vi "CAN_initialize2.vi"() -> (0 "Array 2":errorcluster[](array[cluster]), 1 "Array":refnum<class "sbCANopenBaseClass.lvclass">[](array[class]), 2 "Motors to use":bool[](array[boolean]))   [LabVIEW 2024]
uses:
  <vilib>/addons/Maxon Motor/EPOS2 CANopen/EPOS2 Library.lvlib
  <vilib>/addons/Maxon Motor/EPOS2 CANopen/EPOS2 Support Files/Polymorphic SubVIs/Config/EPOS2 Current Mode Configure.vi
  <vilib>/addons/Maxon Motor/EPOS2 CANopen/EPOS2 Support Files/Typedefs/EPOS2 Velocity Units.ctl
  <vilib>/addons/Maxon Motor/EPOS2 CANopen/EPOS2 Support Files/Typedefs/EPOS2 Config Data Input Current.ctl
  <vilib>/addons/Maxon Motor/EPOS2 CANopen/CANopen/CANopen IndCom Interface/sdCANopenIndCom.lvclass
  <vilib>/addons/Maxon Motor/EPOS2 CANopen/CANopen/sbCANopenBaseClass.lvclass
panel:
  out "MU":i32[](array[numeric])
  out "size(s) 3":i32
  out "appended array 2":refnum<class "sbCANopenBaseClass.lvclass">[](array[class])
  out "size(s)":i32
  out "size(s) 2":i32
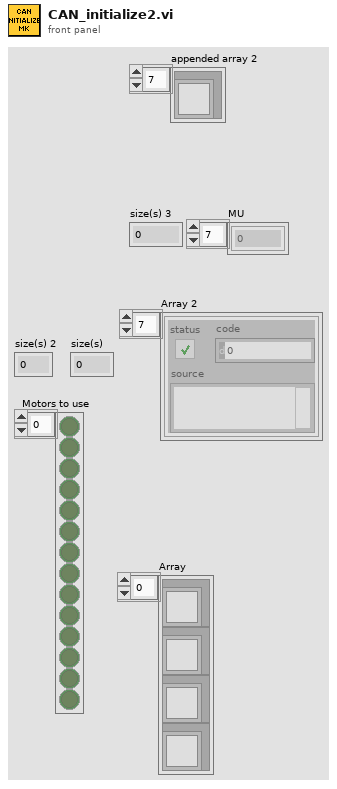
[diagram p1: front panel]
types:
  T1 = typedef "EPOS2 Library.lvlib/EPOS2 Config Data Input Current.ctl" = cluster{"Velocity Units":T2, "Max Velocity":i32}
  T2 = typedef "EPOS2 Library.lvlib/EPOS2 Velocity Units.ctl" = i8
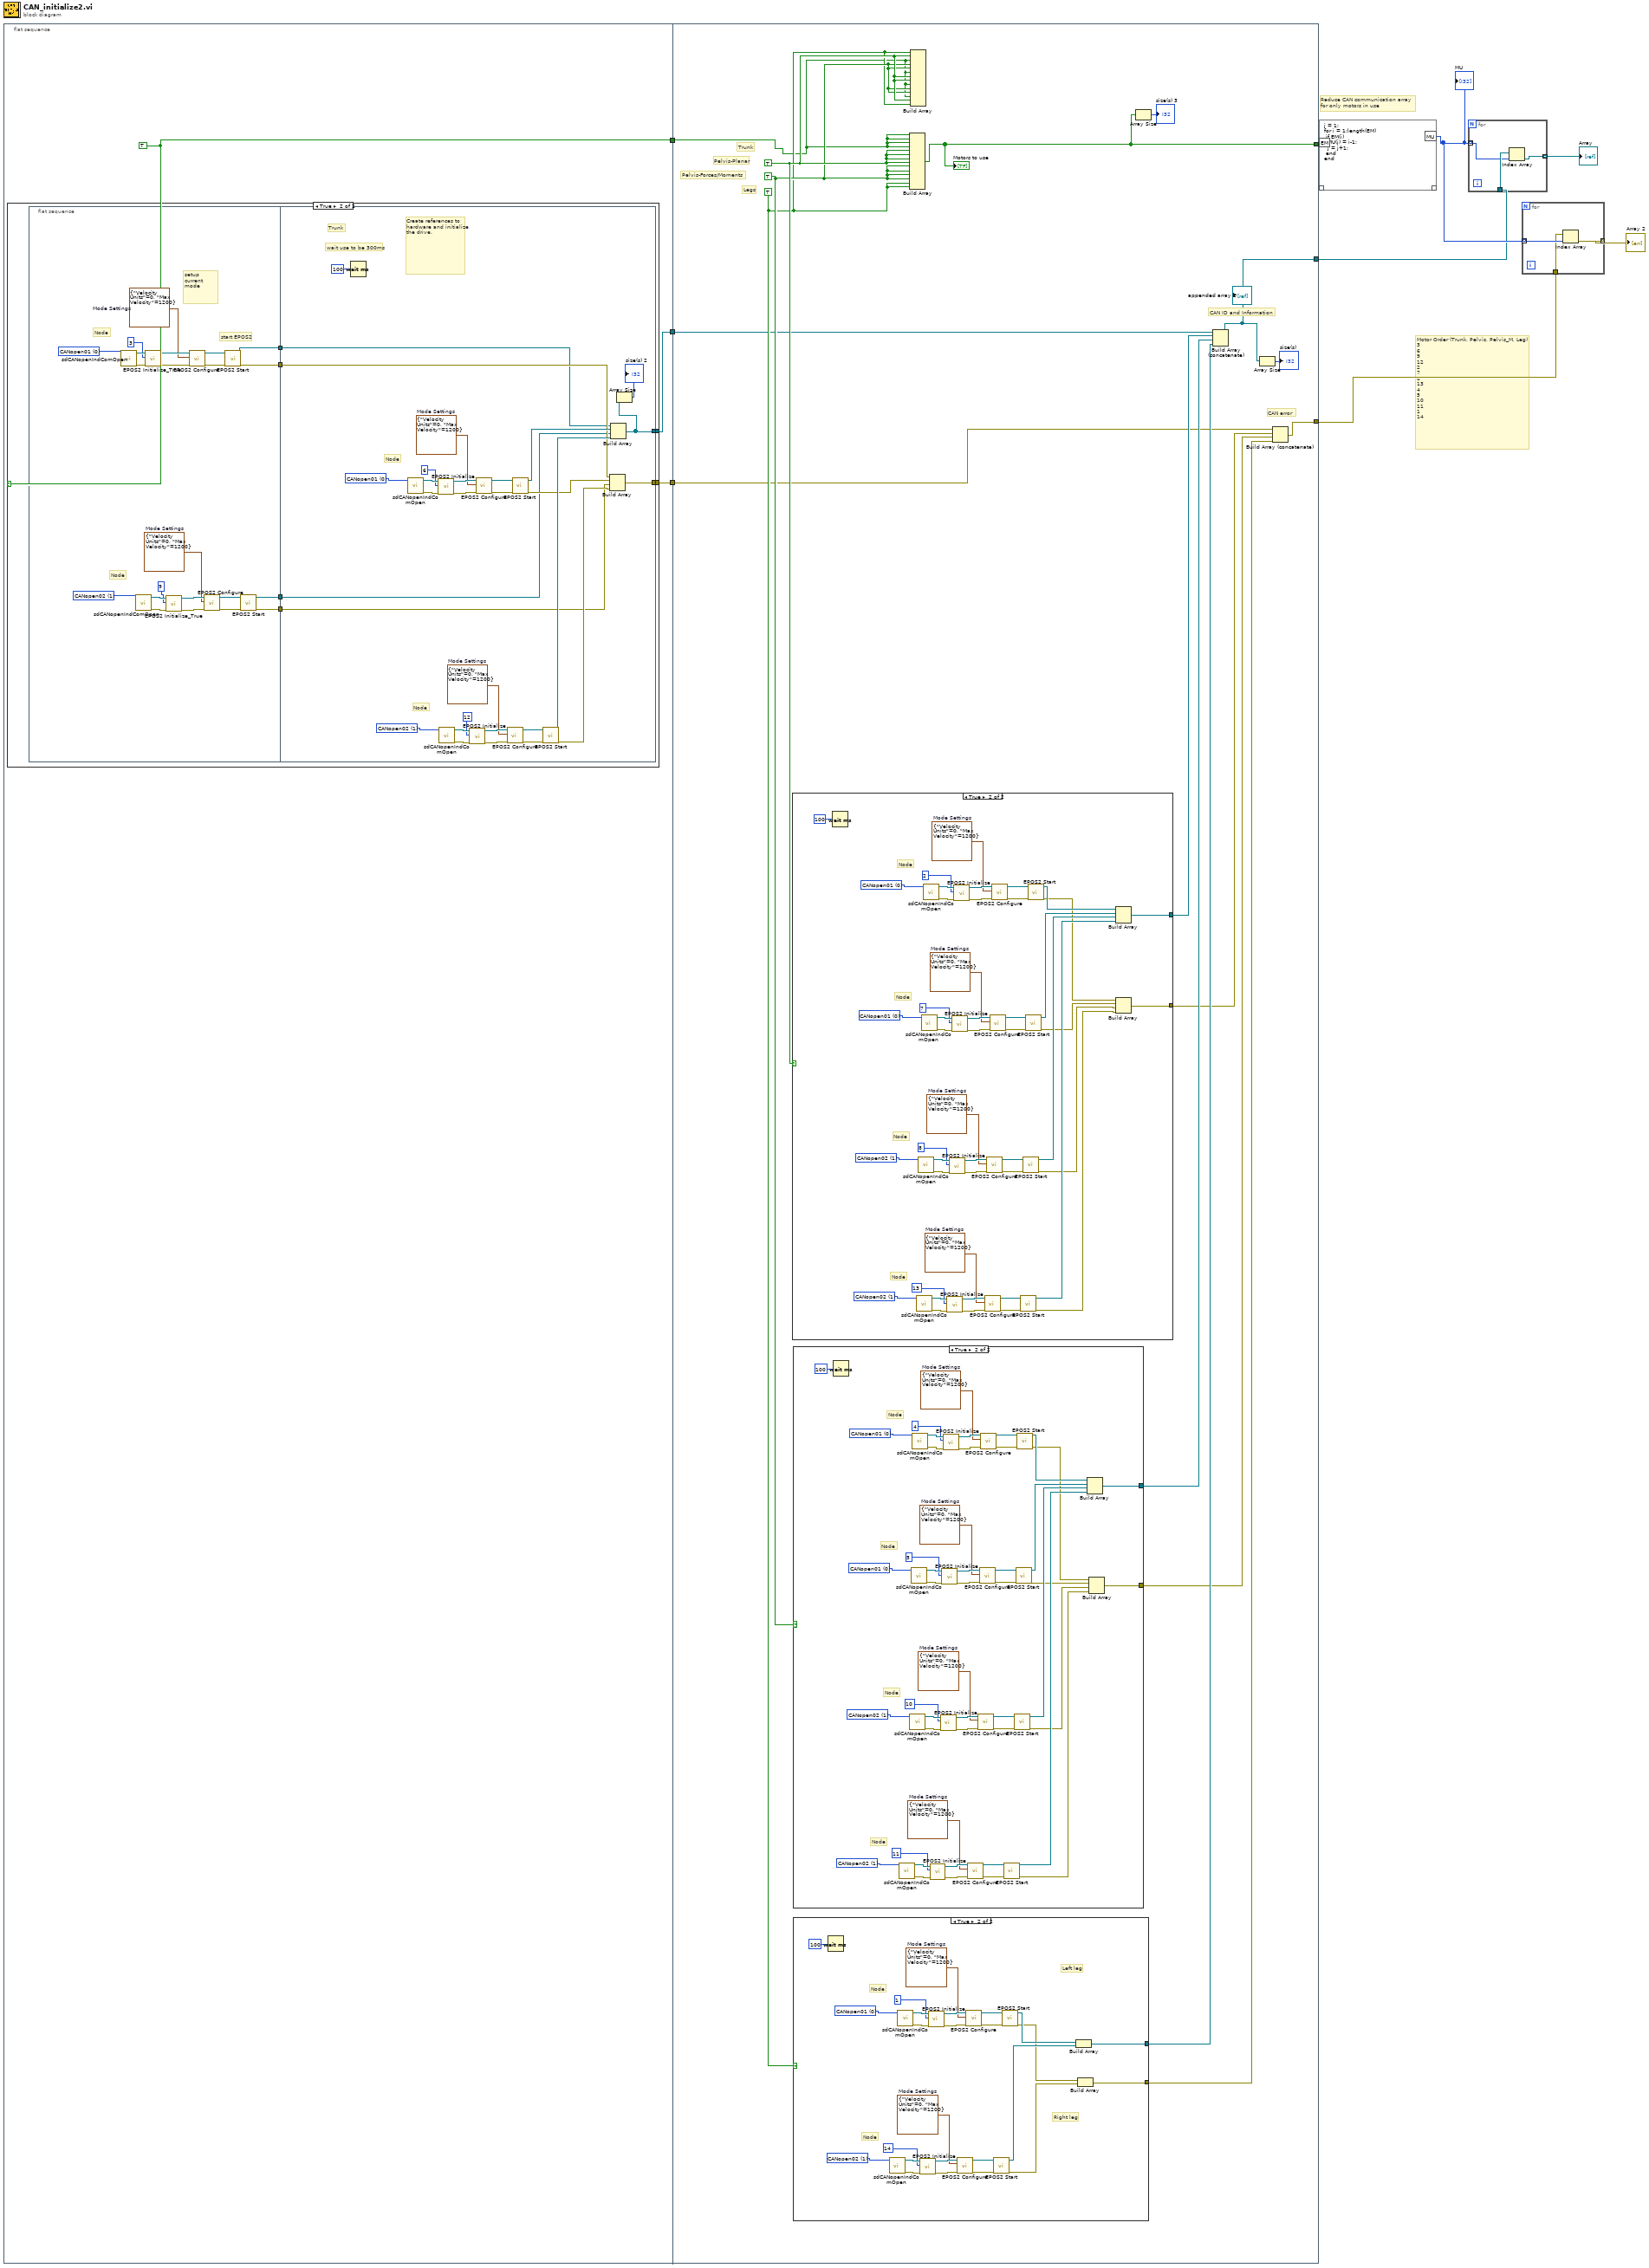
[diagram p0: block diagram]
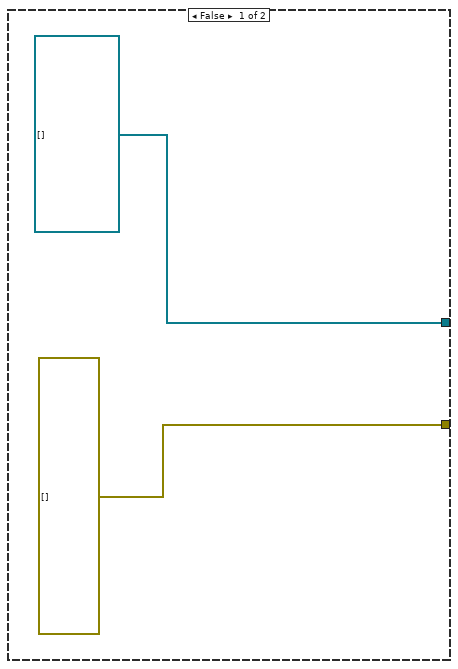
[diagram p2: hidden frame]
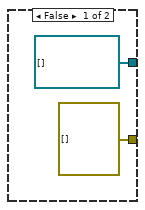
[diagram p3: hidden frame]
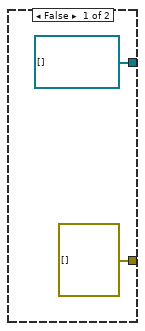
[diagram p4: hidden frame]
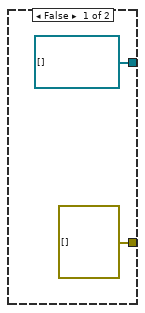
[diagram p5: hidden frame]
diagram:
  # "Motor Order (Trunk, Pelvis, Pelvis_M, Leg)\n3\n6\n9\n12\n2\n7\n8\n13\n4\n5\n10\n11\n1\n14"
  # "Reduce CAN communication array \nfor only motors in use"
  n1 = flat-sequence {
    tunnel: [w10] -> w3
    tunnel: [w12] -> w2
    tunnel: [w11] -> w1
    tunnel: [w82] -> w6
    tunnel: [w81] -> w5
    tunnel: [w76] -> w4
    tunnel: w3 -> [w75]
    tunnel: w2 -> [w74]
    tunnel: w1 -> [w73]
    frame #0 {
      w10 = TRUE
      n2 = case shown="True" w10 {
        tunnel: [refnum<class "sbCANopenBaseClass.lvclass">[] [] w20] -> w12
        tunnel: [errorcluster[] [] w19] -> w11
        frame False {
        }
        frame True {
          n3 = flat-sequence {
            tunnel: [w33] -> w18
            tunnel: [w32] -> w17
            tunnel: [w22] -> w16
            tunnel: [w21] -> w15
            tunnel: [w48] -> w20
            tunnel: [w47] -> w19
            tunnel: w18 -> [w46]
            tunnel: w17 -> [w45]
            tunnel: w16 -> [w44]
            tunnel: w15 -> [w43]
            frame #0 {
              w24 = u32 1 items=["CANopen01", "CANopen02", "CANopen03", "CANopen04", "CANopen05", "CANopen06", "CANopen07", "CANopen08", "CANopen09", "CANopen10", "CANopen11", "CANopen12", "CANopen13", "CANopen14", "CANopen15", "CANopen16", "CANopen17", "CANopen18", "CANopen19", "CANopen20", "CANopen21", "CANopen22", "CANopen23", "CANopen24", "CANopen25", "CANopen26", "CANopen27", "CANopen28", "CANopen29", "CANopen30", "CANopen31", "CANopen32"] ("Interface Name")
              w23 = T1 {"Velocity Units"=0, "Max Velocity"=1200}  # Mode Settings
              w35 = u32 0 items=["CANopen01", "CANopen02", "CANopen03", "CANopen04", "CANopen05", "CANopen06", "CANopen07", "CANopen08", "CANopen09", "CANopen10", "CANopen11", "CANopen12", "CANopen13", "CANopen14", "CANopen15", "CANopen16", "CANopen17", "CANopen18", "CANopen19", "CANopen20", "CANopen21", "CANopen22", "CANopen23", "CANopen24", "CANopen25", "CANopen26", "CANopen27", "CANopen28", "CANopen29", "CANopen30", "CANopen31", "CANopen32"] ("Interface Name")
              w34 = T1 {"Velocity Units"=0, "Max Velocity"=1200}  # Mode Settings
              # "Node"
              # "Node"
              # "start EPOS2"
              # "setup current mode"
              n4 = call <vilib>:"sdCANopenIndComOpen.vi"("Interface Name"=w35) -> ("error out"=w38:errorcluster, "SD CANopen Comm out"=w42:refnum<class "sbCANopenBaseClass.lvclass">)  [unwired: 9 in]
              n5 = call <vilib>:"sdCANopenIndComOpen.vi"("Interface Name"=w24) -> ("error out"=w27:errorcluster, "SD CANopen Comm out"=w31:refnum<class "sbCANopenBaseClass.lvclass">)  [unwired: 9 in]
              n6 = call <vilib>:"EPOS2 Initialize_True.vi"("error in"=w38, "Node ID"=u8 3, "CAN Session In"=w42) -> ("error out"=w37:errorcluster, "CANopen Session Out"=w40:refnum<class "sbCANopenBaseClass.lvclass">)  [unwired: 7 in]
              n7 = call <vilib>:"EPOS2 Initialize_True.vi"("error in"=w27, "Node ID"=u8 9, "CAN Session In"=w31) -> ("error out"=w26:errorcluster, "CANopen Session Out"=w29:refnum<class "sbCANopenBaseClass.lvclass">)  [unwired: 7 in]
              n8 = call-poly <vilib>:"EPOS2 Configure.vi"("error in"=w37, "Mode Settings"=w34, "CANopen Session In"=w40) -> ("error out"=w39:errorcluster, "CANopen Session Out"=w41:refnum<class "sbCANopenBaseClass.lvclass">)  [unwired: 7 in]
              n9 = call-poly <vilib>:"EPOS2 Configure.vi"("error in"=w26, "Mode Settings"=w23, "CANopen Session In"=w29) -> ("error out"=w28:errorcluster, "CANopen Session Out"=w30:refnum<class "sbCANopenBaseClass.lvclass">)  [unwired: 7 in]
              n10 = call <vilib>:"EPOS2 Start.vi"("error in"=w39, "CANopen Session In"=w41) -> ("error out"=w33:errorcluster, "CANopen Session Out"=w32:refnum<class "sbCANopenBaseClass.lvclass">)  [unwired: 8 in]
              n11 = call <vilib>:"EPOS2 Start.vi"("error in"=w28, "CANopen Session In"=w30) -> ("error out"=w22:errorcluster, "CANopen Session Out"=w21:refnum<class "sbCANopenBaseClass.lvclass">)  [unwired: 8 in]
            }
            frame #1 {
              w58 = u32 1 items=["CANopen01", "CANopen02", "CANopen03", "CANopen04", "CANopen05", "CANopen06", "CANopen07", "CANopen08", "CANopen09", "CANopen10", "CANopen11", "CANopen12", "CANopen13", "CANopen14", "CANopen15", "CANopen16", "CANopen17", "CANopen18", "CANopen19", "CANopen20", "CANopen21", "CANopen22", "CANopen23", "CANopen24", "CANopen25", "CANopen26", "CANopen27", "CANopen28", "CANopen29", "CANopen30", "CANopen31", "CANopen32"] ("Interface Name")
              w59 = T1 {"Velocity Units"=0, "Max Velocity"=1200}  # Mode Settings
              w66 = u32 0 items=["CANopen01", "CANopen02", "CANopen03", "CANopen04", "CANopen05", "CANopen06", "CANopen07", "CANopen08", "CANopen09", "CANopen10", "CANopen11", "CANopen12", "CANopen13", "CANopen14", "CANopen15", "CANopen16", "CANopen17", "CANopen18", "CANopen19", "CANopen20", "CANopen21", "CANopen22", "CANopen23", "CANopen24", "CANopen25", "CANopen26", "CANopen27", "CANopen28", "CANopen29", "CANopen30", "CANopen31", "CANopen32"] ("Interface Name")
              w67 = T1 {"Velocity Units"=0, "Max Velocity"=1200}  # Mode Settings
              # "wait use to be 300ms"
              # "Node"
              # "Node"
              # "Trunk"
              # "Create references to hardware and initialize the drive."
              n12 = Wait (ms)(milliseconds to wait=u32 100) -> ()  [unwired: 1 out]
              n13 = call <vilib>:"sdCANopenIndComOpen.vi"("Interface Name"=w66) -> ("error out"=w71:errorcluster, "SD CANopen Comm out"=w65:refnum<class "sbCANopenBaseClass.lvclass">)  [unwired: 9 in]
              n14 = call <vilib>:"EPOS2 Initialize.vi"("error in"=w71, "Node ID"=u8 6, "CAN Session In"=w65) -> ("error out"=w72:errorcluster, "CANopen Session Out"=w69:refnum<class "sbCANopenBaseClass.lvclass">)  [unwired: 1 in, 6 out]
              n15 = call <vilib>:"sdCANopenIndComOpen.vi"("Interface Name"=w58) -> ("error out"=w63:errorcluster, "SD CANopen Comm out"=w57:refnum<class "sbCANopenBaseClass.lvclass">)  [unwired: 9 in]
              n16 = call <vilib>:"EPOS2 Initialize.vi"("error in"=w63, "Node ID"=u8 12, "CAN Session In"=w57) -> ("error out"=w64:errorcluster, "CANopen Session Out"=w61:refnum<class "sbCANopenBaseClass.lvclass">)  [unwired: 1 in, 6 out]
              n17 = call-poly <vilib>:"EPOS2 Configure.vi"("error in"=w72, "Mode Settings"=w67, "CANopen Session In"=w69) -> ("error out"=w70:errorcluster, "CANopen Session Out"=w68:refnum<class "sbCANopenBaseClass.lvclass">)  [unwired: 7 in]
              n18 = call-poly <vilib>:"EPOS2 Configure.vi"("error in"=w64, "Mode Settings"=w59, "CANopen Session In"=w61) -> ("error out"=w62:errorcluster, "CANopen Session Out"=w60:refnum<class "sbCANopenBaseClass.lvclass">)  [unwired: 7 in]
              n19 = call <vilib>:"EPOS2 Start.vi"("error in"=w70, "CANopen Session In"=w68) -> ("error out"=w54:errorcluster, "CANopen Session Out"=w56:refnum<class "sbCANopenBaseClass.lvclass">)  [unwired: 8 in]
              n20 = call <vilib>:"EPOS2 Start.vi"("error in"=w62, "CANopen Session In"=w60) -> ("error out"=w53:errorcluster, "CANopen Session Out"=w55:refnum<class "sbCANopenBaseClass.lvclass">)  [unwired: 8 in]
              n21 = Build Array(w46, w54, w44, w53) -> (w47:errorcluster[])
              n22 = Build Array(w45, w56, w43, w55) -> (w48:refnum<class "sbCANopenBaseClass.lvclass">[])
              n23 = Array Size(array=w48) -> (size(s)=→"size(s) 2":i32)
            }
          }
        }
      }
    }
    frame #1 {
      w77 = TRUE
      w78 = TRUE
      w79 = TRUE
      # "CAN error"
      # "CAN ID and Information"
      # "Legs"
      # "Pelvis-Forces/Moments"
      # "Pelvis-Planar"
      # "Trunk"
      n24 = case shown="True" w79 {
        tunnel: [refnum<class "sbCANopenBaseClass.lvclass">[] [] w178] -> w89
        tunnel: [errorcluster[] [] w173] -> w86
        frame False {
        }
        frame True {
          w184 = u32 1 items=["CANopen01", "CANopen02", "CANopen03", "CANopen04", "CANopen05", "CANopen06", "CANopen07", "CANopen08", "CANopen09", "CANopen10", "CANopen11", "CANopen12", "CANopen13", "CANopen14", "CANopen15", "CANopen16", "CANopen17", "CANopen18", "CANopen19", "CANopen20", "CANopen21", "CANopen22", "CANopen23", "CANopen24", "CANopen25", "CANopen26", "CANopen27", "CANopen28", "CANopen29", "CANopen30", "CANopen31", "CANopen32"] ("Interface Name")
          w185 = T1 {"Velocity Units"=0, "Max Velocity"=1200}  # Mode Settings
          w192 = u32 1 items=["CANopen01", "CANopen02", "CANopen03", "CANopen04", "CANopen05", "CANopen06", "CANopen07", "CANopen08", "CANopen09", "CANopen10", "CANopen11", "CANopen12", "CANopen13", "CANopen14", "CANopen15", "CANopen16", "CANopen17", "CANopen18", "CANopen19", "CANopen20", "CANopen21", "CANopen22", "CANopen23", "CANopen24", "CANopen25", "CANopen26", "CANopen27", "CANopen28", "CANopen29", "CANopen30", "CANopen31", "CANopen32"] ("Interface Name")
          w193 = T1 {"Velocity Units"=0, "Max Velocity"=1200}  # Mode Settings
          w200 = u32 0 items=["CANopen01", "CANopen02", "CANopen03", "CANopen04", "CANopen05", "CANopen06", "CANopen07", "CANopen08", "CANopen09", "CANopen10", "CANopen11", "CANopen12", "CANopen13", "CANopen14", "CANopen15", "CANopen16", "CANopen17", "CANopen18", "CANopen19", "CANopen20", "CANopen21", "CANopen22", "CANopen23", "CANopen24", "CANopen25", "CANopen26", "CANopen27", "CANopen28", "CANopen29", "CANopen30", "CANopen31", "CANopen32"] ("Interface Name")
          w201 = T1 {"Velocity Units"=0, "Max Velocity"=1200}  # Mode Settings
          w208 = u32 0 items=["CANopen01", "CANopen02", "CANopen03", "CANopen04", "CANopen05", "CANopen06", "CANopen07", "CANopen08", "CANopen09", "CANopen10", "CANopen11", "CANopen12", "CANopen13", "CANopen14", "CANopen15", "CANopen16", "CANopen17", "CANopen18", "CANopen19", "CANopen20", "CANopen21", "CANopen22", "CANopen23", "CANopen24", "CANopen25", "CANopen26", "CANopen27", "CANopen28", "CANopen29", "CANopen30", "CANopen31", "CANopen32"] ("Interface Name")
          w209 = T1 {"Velocity Units"=0, "Max Velocity"=1200}  # Mode Settings
          # "Node"
          # "Node"
          # "Node"
          # "Node"
          n25 = Wait (ms)(milliseconds to wait=u32 100) -> ()  [unwired: 1 out]
          n26 = call <vilib>:"sdCANopenIndComOpen.vi"("Interface Name"=w184) -> ("error out"=w189:errorcluster, "SD CANopen Comm out"=w183:refnum<class "sbCANopenBaseClass.lvclass">)  [unwired: 9 in]
          n27 = call <vilib>:"sdCANopenIndComOpen.vi"("Interface Name"=w192) -> ("error out"=w197:errorcluster, "SD CANopen Comm out"=w191:refnum<class "sbCANopenBaseClass.lvclass">)  [unwired: 9 in]
          n28 = call <vilib>:"sdCANopenIndComOpen.vi"("Interface Name"=w200) -> ("error out"=w205:errorcluster, "SD CANopen Comm out"=w199:refnum<class "sbCANopenBaseClass.lvclass">)  [unwired: 9 in]
          n29 = call <vilib>:"sdCANopenIndComOpen.vi"("Interface Name"=w208) -> ("error out"=w213:errorcluster, "SD CANopen Comm out"=w207:refnum<class "sbCANopenBaseClass.lvclass">)  [unwired: 9 in]
          n30 = call <vilib>:"EPOS2 Initialize.vi"("error in"=w189, "Node ID"=u8 13, "CAN Session In"=w183) -> ("error out"=w190:errorcluster, "CANopen Session Out"=w187:refnum<class "sbCANopenBaseClass.lvclass">)  [unwired: 1 in, 6 out]
          n31 = call <vilib>:"EPOS2 Initialize.vi"("error in"=w197, "Node ID"=u8 8, "CAN Session In"=w191) -> ("error out"=w198:errorcluster, "CANopen Session Out"=w195:refnum<class "sbCANopenBaseClass.lvclass">)  [unwired: 1 in, 6 out]
          n32 = call <vilib>:"EPOS2 Initialize.vi"("error in"=w205, "Node ID"=u8 7, "CAN Session In"=w199) -> ("error out"=w206:errorcluster, "CANopen Session Out"=w203:refnum<class "sbCANopenBaseClass.lvclass">)  [unwired: 1 in, 6 out]
          n33 = call <vilib>:"EPOS2 Initialize.vi"("error in"=w213, "Node ID"=u8 2, "CAN Session In"=w207) -> ("error out"=w214:errorcluster, "CANopen Session Out"=w211:refnum<class "sbCANopenBaseClass.lvclass">)  [unwired: 1 in, 6 out]
          n34 = call-poly <vilib>:"EPOS2 Configure.vi"("error in"=w190, "Mode Settings"=w185, "CANopen Session In"=w187) -> ("error out"=w188:errorcluster, "CANopen Session Out"=w186:refnum<class "sbCANopenBaseClass.lvclass">)  [unwired: 7 in]
          n35 = call-poly <vilib>:"EPOS2 Configure.vi"("error in"=w198, "Mode Settings"=w193, "CANopen Session In"=w195) -> ("error out"=w196:errorcluster, "CANopen Session Out"=w194:refnum<class "sbCANopenBaseClass.lvclass">)  [unwired: 7 in]
          n36 = call-poly <vilib>:"EPOS2 Configure.vi"("error in"=w206, "Mode Settings"=w201, "CANopen Session In"=w203) -> ("error out"=w204:errorcluster, "CANopen Session Out"=w202:refnum<class "sbCANopenBaseClass.lvclass">)  [unwired: 7 in]
          n37 = call-poly <vilib>:"EPOS2 Configure.vi"("error in"=w214, "Mode Settings"=w209, "CANopen Session In"=w211) -> ("error out"=w212:errorcluster, "CANopen Session Out"=w210:refnum<class "sbCANopenBaseClass.lvclass">)  [unwired: 7 in]
          n38 = call <vilib>:"EPOS2 Start.vi"("error in"=w188, "CANopen Session In"=w186) -> ("error out"=w174:errorcluster, "CANopen Session Out"=w179:refnum<class "sbCANopenBaseClass.lvclass">)  [unwired: 8 in]
          n39 = call <vilib>:"EPOS2 Start.vi"("error in"=w196, "CANopen Session In"=w194) -> ("error out"=w175:errorcluster, "CANopen Session Out"=w180:refnum<class "sbCANopenBaseClass.lvclass">)  [unwired: 8 in]
          n40 = call <vilib>:"EPOS2 Start.vi"("error in"=w204, "CANopen Session In"=w202) -> ("error out"=w176:errorcluster, "CANopen Session Out"=w181:refnum<class "sbCANopenBaseClass.lvclass">)  [unwired: 8 in]
          n41 = call <vilib>:"EPOS2 Start.vi"("error in"=w212, "CANopen Session In"=w210) -> ("error out"=w177:errorcluster, "CANopen Session Out"=w182:refnum<class "sbCANopenBaseClass.lvclass">)  [unwired: 8 in]
          n42 = Build Array(w182, w181, w180, w179) -> (w178:refnum<class "sbCANopenBaseClass.lvclass">[])
          n43 = Build Array(w177, w176, w175, w174) -> (w173:errorcluster[])
        }
      }
      n44 = case shown="True" w78 {
        tunnel: [refnum<class "sbCANopenBaseClass.lvclass">[] [] w129] -> w88
        tunnel: [errorcluster[] [] w124] -> w85
        frame False {
        }
        frame True {
          w135 = u32 1 items=["CANopen01", "CANopen02", "CANopen03", "CANopen04", "CANopen05", "CANopen06", "CANopen07", "CANopen08", "CANopen09", "CANopen10", "CANopen11", "CANopen12", "CANopen13", "CANopen14", "CANopen15", "CANopen16", "CANopen17", "CANopen18", "CANopen19", "CANopen20", "CANopen21", "CANopen22", "CANopen23", "CANopen24", "CANopen25", "CANopen26", "CANopen27", "CANopen28", "CANopen29", "CANopen30", "CANopen31", "CANopen32"] ("Interface Name")
          w136 = T1 {"Velocity Units"=0, "Max Velocity"=1200}  # Mode Settings
          w143 = u32 1 items=["CANopen01", "CANopen02", "CANopen03", "CANopen04", "CANopen05", "CANopen06", "CANopen07", "CANopen08", "CANopen09", "CANopen10", "CANopen11", "CANopen12", "CANopen13", "CANopen14", "CANopen15", "CANopen16", "CANopen17", "CANopen18", "CANopen19", "CANopen20", "CANopen21", "CANopen22", "CANopen23", "CANopen24", "CANopen25", "CANopen26", "CANopen27", "CANopen28", "CANopen29", "CANopen30", "CANopen31", "CANopen32"] ("Interface Name")
          w144 = T1 {"Velocity Units"=0, "Max Velocity"=1200}  # Mode Settings
          w151 = u32 0 items=["CANopen01", "CANopen02", "CANopen03", "CANopen04", "CANopen05", "CANopen06", "CANopen07", "CANopen08", "CANopen09", "CANopen10", "CANopen11", "CANopen12", "CANopen13", "CANopen14", "CANopen15", "CANopen16", "CANopen17", "CANopen18", "CANopen19", "CANopen20", "CANopen21", "CANopen22", "CANopen23", "CANopen24", "CANopen25", "CANopen26", "CANopen27", "CANopen28", "CANopen29", "CANopen30", "CANopen31", "CANopen32"] ("Interface Name")
          w152 = T1 {"Velocity Units"=0, "Max Velocity"=1200}  # Mode Settings
          w159 = u32 0 items=["CANopen01", "CANopen02", "CANopen03", "CANopen04", "CANopen05", "CANopen06", "CANopen07", "CANopen08", "CANopen09", "CANopen10", "CANopen11", "CANopen12", "CANopen13", "CANopen14", "CANopen15", "CANopen16", "CANopen17", "CANopen18", "CANopen19", "CANopen20", "CANopen21", "CANopen22", "CANopen23", "CANopen24", "CANopen25", "CANopen26", "CANopen27", "CANopen28", "CANopen29", "CANopen30", "CANopen31", "CANopen32"] ("Interface Name")
          w160 = T1 {"Velocity Units"=0, "Max Velocity"=1200}  # Mode Settings
          # "Node"
          # "Node"
          # "Node"
          # "Node"
          n45 = Wait (ms)(milliseconds to wait=u32 100) -> ()  [unwired: 1 out]
          n46 = call <vilib>:"sdCANopenIndComOpen.vi"("Interface Name"=w135) -> ("error out"=w140:errorcluster, "SD CANopen Comm out"=w134:refnum<class "sbCANopenBaseClass.lvclass">)  [unwired: 9 in]
          n47 = call <vilib>:"sdCANopenIndComOpen.vi"("Interface Name"=w143) -> ("error out"=w148:errorcluster, "SD CANopen Comm out"=w142:refnum<class "sbCANopenBaseClass.lvclass">)  [unwired: 9 in]
          n48 = call <vilib>:"sdCANopenIndComOpen.vi"("Interface Name"=w151) -> ("error out"=w156:errorcluster, "SD CANopen Comm out"=w150:refnum<class "sbCANopenBaseClass.lvclass">)  [unwired: 9 in]
          n49 = call <vilib>:"sdCANopenIndComOpen.vi"("Interface Name"=w159) -> ("error out"=w164:errorcluster, "SD CANopen Comm out"=w158:refnum<class "sbCANopenBaseClass.lvclass">)  [unwired: 9 in]
          n50 = call <vilib>:"EPOS2 Initialize.vi"("error in"=w140, "Node ID"=u8 11, "CAN Session In"=w134) -> ("error out"=w141:errorcluster, "CANopen Session Out"=w138:refnum<class "sbCANopenBaseClass.lvclass">)  [unwired: 1 in, 6 out]
          n51 = call <vilib>:"EPOS2 Initialize.vi"("error in"=w148, "Node ID"=u8 10, "CAN Session In"=w142) -> ("error out"=w149:errorcluster, "CANopen Session Out"=w146:refnum<class "sbCANopenBaseClass.lvclass">)  [unwired: 1 in, 6 out]
          n52 = call <vilib>:"EPOS2 Initialize.vi"("error in"=w156, "Node ID"=u8 5, "CAN Session In"=w150) -> ("error out"=w157:errorcluster, "CANopen Session Out"=w154:refnum<class "sbCANopenBaseClass.lvclass">)  [unwired: 1 in, 6 out]
          n53 = call <vilib>:"EPOS2 Initialize.vi"("error in"=w164, "Node ID"=u8 4, "CAN Session In"=w158) -> ("error out"=w165:errorcluster, "CANopen Session Out"=w162:refnum<class "sbCANopenBaseClass.lvclass">)  [unwired: 1 in, 6 out]
          n54 = call-poly <vilib>:"EPOS2 Configure.vi"("error in"=w141, "Mode Settings"=w136, "CANopen Session In"=w138) -> ("error out"=w139:errorcluster, "CANopen Session Out"=w137:refnum<class "sbCANopenBaseClass.lvclass">)  [unwired: 7 in]
          n55 = call-poly <vilib>:"EPOS2 Configure.vi"("error in"=w149, "Mode Settings"=w144, "CANopen Session In"=w146) -> ("error out"=w147:errorcluster, "CANopen Session Out"=w145:refnum<class "sbCANopenBaseClass.lvclass">)  [unwired: 7 in]
          n56 = call-poly <vilib>:"EPOS2 Configure.vi"("error in"=w157, "Mode Settings"=w152, "CANopen Session In"=w154) -> ("error out"=w155:errorcluster, "CANopen Session Out"=w153:refnum<class "sbCANopenBaseClass.lvclass">)  [unwired: 7 in]
          n57 = call-poly <vilib>:"EPOS2 Configure.vi"("error in"=w165, "Mode Settings"=w160, "CANopen Session In"=w162) -> ("error out"=w163:errorcluster, "CANopen Session Out"=w161:refnum<class "sbCANopenBaseClass.lvclass">)  [unwired: 7 in]
          n58 = call <vilib>:"EPOS2 Start.vi"("error in"=w139, "CANopen Session In"=w137) -> ("error out"=w125:errorcluster, "CANopen Session Out"=w130:refnum<class "sbCANopenBaseClass.lvclass">)  [unwired: 8 in]
          n59 = call <vilib>:"EPOS2 Start.vi"("error in"=w147, "CANopen Session In"=w145) -> ("error out"=w126:errorcluster, "CANopen Session Out"=w131:refnum<class "sbCANopenBaseClass.lvclass">)  [unwired: 8 in]
          n60 = call <vilib>:"EPOS2 Start.vi"("error in"=w155, "CANopen Session In"=w153) -> ("error out"=w127:errorcluster, "CANopen Session Out"=w132:refnum<class "sbCANopenBaseClass.lvclass">)  [unwired: 8 in]
          n61 = call <vilib>:"EPOS2 Start.vi"("error in"=w163, "CANopen Session In"=w161) -> ("error out"=w128:errorcluster, "CANopen Session Out"=w133:refnum<class "sbCANopenBaseClass.lvclass">)  [unwired: 8 in]
          n62 = Build Array(w133, w132, w131, w130) -> (w129:refnum<class "sbCANopenBaseClass.lvclass">[])
          n63 = Build Array(w128, w127, w126, w125) -> (w124:errorcluster[])
        }
      }
      n64 = case shown="True" w77 {
        tunnel: [refnum<class "sbCANopenBaseClass.lvclass">[] [] w98] -> w87
        tunnel: [errorcluster[] [] w95] -> w84
        frame False {
        }
        frame True {
          w102 = u32 1 items=["CANopen01", "CANopen02", "CANopen03", "CANopen04", "CANopen05", "CANopen06", "CANopen07", "CANopen08", "CANopen09", "CANopen10", "CANopen11", "CANopen12", "CANopen13", "CANopen14", "CANopen15", "CANopen16", "CANopen17", "CANopen18", "CANopen19", "CANopen20", "CANopen21", "CANopen22", "CANopen23", "CANopen24", "CANopen25", "CANopen26", "CANopen27", "CANopen28", "CANopen29", "CANopen30", "CANopen31", "CANopen32"] ("Interface Name")
          w103 = T1 {"Velocity Units"=0, "Max Velocity"=1200}  # Mode Settings
          w110 = u32 0 items=["CANopen01", "CANopen02", "CANopen03", "CANopen04", "CANopen05", "CANopen06", "CANopen07", "CANopen08", "CANopen09", "CANopen10", "CANopen11", "CANopen12", "CANopen13", "CANopen14", "CANopen15", "CANopen16", "CANopen17", "CANopen18", "CANopen19", "CANopen20", "CANopen21", "CANopen22", "CANopen23", "CANopen24", "CANopen25", "CANopen26", "CANopen27", "CANopen28", "CANopen29", "CANopen30", "CANopen31", "CANopen32"] ("Interface Name")
          w111 = T1 {"Velocity Units"=0, "Max Velocity"=1200}  # Mode Settings
          # "Right leg"
          # "Left leg"
          # "Node"
          # "Node"
          n65 = Wait (ms)(milliseconds to wait=u32 100) -> ()  [unwired: 1 out]
          n66 = call <vilib>:"sdCANopenIndComOpen.vi"("Interface Name"=w102) -> ("error out"=w107:errorcluster, "SD CANopen Comm out"=w101:refnum<class "sbCANopenBaseClass.lvclass">)  [unwired: 9 in]
          n67 = call <vilib>:"sdCANopenIndComOpen.vi"("Interface Name"=w110) -> ("error out"=w115:errorcluster, "SD CANopen Comm out"=w109:refnum<class "sbCANopenBaseClass.lvclass">)  [unwired: 9 in]
          n68 = call <vilib>:"EPOS2 Initialize.vi"("error in"=w107, "Node ID"=u8 14, "CAN Session In"=w101) -> ("error out"=w108:errorcluster, "CANopen Session Out"=w105:refnum<class "sbCANopenBaseClass.lvclass">)  [unwired: 1 in, 6 out]
          n69 = call <vilib>:"EPOS2 Initialize.vi"("error in"=w115, "Node ID"=u8 1, "CAN Session In"=w109) -> ("error out"=w116:errorcluster, "CANopen Session Out"=w113:refnum<class "sbCANopenBaseClass.lvclass">)  [unwired: 1 in, 6 out]
          n70 = call-poly <vilib>:"EPOS2 Configure.vi"("error in"=w108, "Mode Settings"=w103, "CANopen Session In"=w105) -> ("error out"=w106:errorcluster, "CANopen Session Out"=w104:refnum<class "sbCANopenBaseClass.lvclass">)  [unwired: 7 in]
          n71 = call-poly <vilib>:"EPOS2 Configure.vi"("error in"=w116, "Mode Settings"=w111, "CANopen Session In"=w113) -> ("error out"=w114:errorcluster, "CANopen Session Out"=w112:refnum<class "sbCANopenBaseClass.lvclass">)  [unwired: 7 in]
          n72 = call <vilib>:"EPOS2 Start.vi"("error in"=w106, "CANopen Session In"=w104) -> ("error out"=w96:errorcluster, "CANopen Session Out"=w99:refnum<class "sbCANopenBaseClass.lvclass">)  [unwired: 8 in]
          n73 = call <vilib>:"EPOS2 Start.vi"("error in"=w114, "CANopen Session In"=w112) -> ("error out"=w97:errorcluster, "CANopen Session Out"=w100:refnum<class "sbCANopenBaseClass.lvclass">)  [unwired: 8 in]
          n74 = Build Array(w100, w99) -> (w98:refnum<class "sbCANopenBaseClass.lvclass">[])
          n75 = Build Array(w97, w96) -> (w95:errorcluster[])
        }
      }
      n76 = Build Array(w75, w75, w75, w75, w79, w79, w79, w79, w78, w78, w78, w78, w77, w77) -> (w76:bool[])
      "Motors to use" <- w76
      n77 = Build Array(w77, w79, w75, w78, w78, w75, w79, w79, w75, w78, w78, w75, w79, w77) -> ()  [unwired: 1 out]
      n78 = Array Size(array=w76) -> (size(s)=→"size(s) 3":i32)
      n79 = Build Array (concatenate)(w74, w89, w88, w87) -> (w81:refnum<class "sbCANopenBaseClass.lvclass">[])
      "appended array 2" <- w81
      n80 = Array Size(array=w81) -> (size(s)=→"size(s)":i32)
      n81 = Build Array (concatenate)(w73, w86, w85, w84) -> (w82:errorcluster[])
    }
  }
  n82 = mathscript code="j = 1;\nfor i = 1:length(EM)\n if EM(i)\n  MU(j) = i-1;\n  j = j+1;\n end\nend"("EM"=w4) -> ("MU"=w9:i32[])  [unwired: 1 in, 1 out]
  "MU" <- w9
  n83 = for {
    tunnel: w9 -> [w216] mode=indexing
    tunnel: w5 -> [w217]
    tunnel: [w215] -> w8 mode=indexing
    n84 = Index Array(array=w217, index=w216) -> (element=w215:refnum<class "sbCANopenBaseClass.lvclass">)
  }
  "Array" <- w8
  n85 = for {
    tunnel: [w220] -> w7 mode=indexing
    tunnel: w9 -> [w219] mode=indexing
    tunnel: w6 -> [w218]
    n86 = Index Array(array=w218, index=w219) -> (element=w220:errorcluster)
  }
  "Array 2" <- w7
